vi "Communication Tests - ServerToClient.vi"(8 "error in (no error)":errorcluster) -> (0 "error out":errorcluster)   [LabVIEW 2017]
uses:
  src/LabVIEW/vi.lib/BenjaminR/Build Farm/Actors/Communication/Connection Listener/Connection Listener Messages/Get Connection List Msg/Get Connection List Msg.lvclass
  C:/Program Files (x86)/National Instruments/LabVIEW 2017/vi.lib/ActorFramework/Reply Msg/Reply Msg.lvclass
  <vilib>/ActorFramework/Message Enqueuer/Message Enqueuer.lvclass
  src/LabVIEW/vi.lib/BenjaminR/Build Farm/Actors/Communication/Connection Listener/Connection Listener/Connection Listener.lvclass/Connection Listener.ctl
  <vilib>/ActorFramework/Reply Msg/Reply Msg.lvclass/Reply Msg.ctl
  <vilib>/ActorFramework/Message Enqueuer/Message Enqueuer.lvclass/Message Enqueuer.ctl
  src/LabVIEW/vi.lib/BenjaminR/Build Farm/Actors/Communication/Connection Listener/Connection Listener Messages/Forward Message Msg/Forward Message Msg.lvclass/Forward Message Msg.ctl
  5aca6dbf-9756-40ca-bd76-575a8f039674.vi
  src/LabVIEW/vi.lib/BenjaminR/Build Farm/Actors/Communication/Connection Listener/Connection Listener/Read Msg Update.vi
  <vilib>/ActorFramework/Message Enqueuer/Enqueue.vi
  src/LabVIEW/vi.lib/BenjaminR/Build Farm/Actors/Communication/Connection Listener/Connection Listener/Connection Listener.lvclass
  C:/Program Files (x86)/National Instruments/LabVIEW 2017/vi.lib/ActorFramework/Actor/Actor.lvclass
  <vilib>/ActorFramework/Reply Msg/Reply Msg.lvclass
  C:/Program Files (x86)/National Instruments/LabVIEW 2017/vi.lib/ActorFramework/Message/Message.lvclass
  src/LabVIEW/vi.lib/BenjaminR/Build Farm/Actors/Communication/Connection Listener/Connection Listener Messages/Forward Message Msg/Forward Message Msg.lvclass
  <vilib>/ActorFramework/Stop Msg/Stop Msg.lvclass
  <vilib>/ActorFramework/Message Priority Queue/Priority Enqueue.vi
  <vilib>/addons/_JKI Toolkits/Caraya/classes/Assert/Assert True.vi
  Support/Communication Clients/Communication Clients/Communication Clients/Communication Clients.lvclass
  <vilib>/ActorFramework/Actor/Actor.lvclass
  <vilib>/addons/_JKI Toolkits/Caraya/classes/Test/Test.lvclass
  <vilib>/addons/_JKI Toolkits/Caraya/classes/Assert/Assert.lvclass
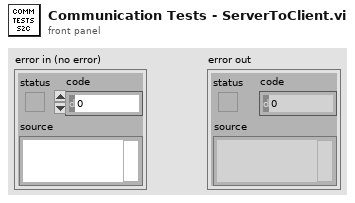
[diagram p1: front panel]
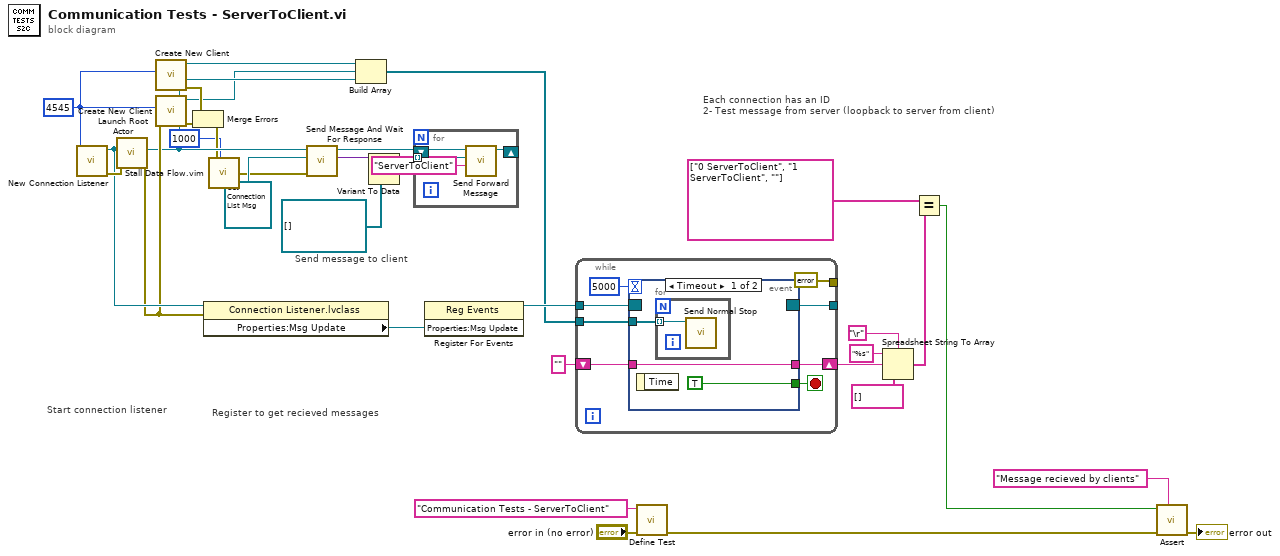
[diagram p0: block diagram]
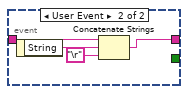
[diagram p2: hidden frame]
diagram:
  w27 = u16 4545 ("Port")
  # "Send message to client"
  # "Register to get recieved messages"
  # "Start connection listener"
  # "Each connection has an ID\n2- Test message from server (loopback to server from client)"
  n1 = call "New Connection Listener.vi"("Port"=w27) -> ("error out"=w33:errorcluster, "Connection Listener out"=w24:refnum<class "Connection Listener.lvclass">)  [unwired: 9 in]
  n2 = call <vilib>:"Launch Root Actor.vi"("error in (no error)"=w33, "Actor"=w24) -> ("error out"=w20:errorcluster, "Actor's Enqueuer"=w13:refnum<class "Message Enqueuer.lvclass">)  [unwired: 8 in]
  n3 = call "Create New Client.vi"("Port"=w27) -> ("error out"=w26:errorcluster, "Message Enqueuer out"=w12:refnum<class "Message Enqueuer.lvclass">)  [unwired: 9 in]
  n4 = call "Create New Client.vi"("error in (no error)"=w20, "Port"=w27) -> ("error out"=w25:errorcluster, "Message Enqueuer out"=w11:refnum<class "Message Enqueuer.lvclass">)  [unwired: 8 in]
  n5 = Merge Errors(w26, w25) -> (w10:errorcluster)
  n6 = property class="Connection Listener.lvclass"(reference=w24, error in=w20) -> ("Properties:Msg Update"=w23:refnum<user-event>)  [unwired: 2 out]
  n7 = call "Stall Data Flow.vim"("value in"=w10, "milliseconds to wait"=u32 1000) -> ("value out"=w2:errorcluster)  [unwired: 1 out]
  n8 = call <vilib>:"Send Message And Wait For Response.vi"("error in (no error)"=w2, "Original Message"=refnum<class "Get Connection List Msg.lvclass"> refnum ("Connection Listener.lvlib:Get Connection List Msg.lvclass"), "Message Enqueuer in"=w13) -> ("Reply"=w31:variant, "Message Enqueuer out"=w29:refnum<class "Message Enqueuer.lvclass">)  [unwired: 5 in, 2 out]
  n9 = Build Array(w12, w11, w13) -> (w9:refnum<class "Message Enqueuer.lvclass">[])
  n10 = Variant To Data(type=refnum<class "Message Enqueuer.lvclass">[] [] ("ConnHandlers"), Variant=w31) -> (data=w28:refnum<class "Message Enqueuer.lvclass">[])  [unwired: 1 in, 1 out]
  n11 = for {
    tunnel: w28 -> [w36] mode=indexing
    shift-right: [w34] -> _
    shift-left: w29 -> [w37]
    n12 = call "Send Forward Message.vi"("Message"="ServerToClient", "Dest Enqueuer"=w36, "Message Enqueuer in"=w37) -> ("Message Enqueuer out"=w34:refnum<class "Message Enqueuer.lvclass">)  [unwired: 7 in, 1 out]
  }
  n13 = register-events(w23) -> (reference out=w22:refnum<event-registration>)  [unwired: 2 in, 1 out]
  n14 = while {
    tunnel: w22 -> [w45]
    shift-right: [w42] -> w19
    shift-left: "" -> [w43]
    tunnel: [w40] -> _
    tunnel: [errorcluster {"status"=FALSE, "code"=0, "source"=""} ("error constant")] -> _
    tunnel: w9 -> [w38]
    stop <- w44 stop-if-true
    n15 = event shown="[0] Timeout" {
      selector: w45 -> [_ _]
      dyn-events: [_ _] -> w40
      timeout: 5000 -> [_ _]
      tunnel: [TRUE ("Discard?") _] -> w44
      tunnel: w43 -> [w48 w53]
      tunnel: [w48 w52] -> w42
      tunnel: w38 -> [w46 _]
      event Timeout {
        n16 = event-data() -> ()  [unwired: 1 in, 1 out]
        n17 = for {
          tunnel: w46 -> [w49] mode=indexing
          n18 = call <vilib>:"Send Normal Stop.vi"("Message Enqueuer"=w49) -> ()  [unwired: 10 in, 1 out]
        }
      }
      event User Event {
        n19 = event-data() -> ("String"=w51:string)  [unwired: 1 in]
        n20 = Concatenate Strings(w53, w51, "\r") -> (w52:string)
      }
    }
  }
  n21 = call <vilib>:"Define Test.vi"("error in (no error)"="error in (no error)", "Label (VI Title)"="Communication Tests - ServerToClient") -> ("error out"=w6:errorcluster)  [unwired: 9 in]
  n22 = Spreadsheet String To Array(delimiter (Tab)="\r", format string="%s", spreadsheet string=w19, array type (2D Dbl)=string[] []) -> (array=w15:string[])
  n23 = Equal?(x=string[] ["0 ServerToClient", "1 ServerToClient", ""] ("array"), y=w15) -> (x = y?=w3:bool)
  n24 = call-poly <vilib>:"Assert.vi"("Label"="Message recieved by clients", "error in (no error)"=w6, "True?"=w3) -> ("error out"=→"error out":errorcluster)  [unwired: 8 in]
